vi "RSZVB Get Power Coeficients Default.vi"(8 "error in (no error)":errorcluster {"code" format="%.0x"}, 11 "VISA session":refnum<visa-resource-name>) -> (0 "error out":errorcluster {"code" format="%.0x"}, 1 "Default Coeficients":bool, 3 "dup VISA session":refnum<visa-resource-name>)   [LabVIEW 2011]
doc: "Returns the state of the default power coefficients for frequency converters R&S ZVA-ZxxxE. \n\nNotes:\n\n(1) This command is available for frequency converters with electronic attenuators R&S ZVA-ZxxxE.\n\nRemote-control command(s):\n[SENSe<Ch>:]FREQuency:CONVersion:DEVice:PCOefficient<Port>:DEFault?>"
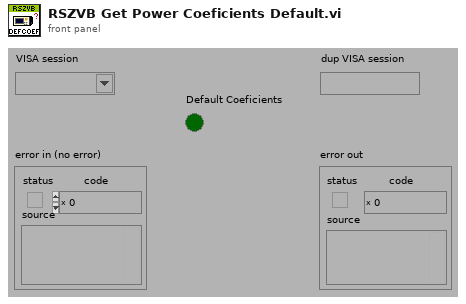
[diagram p1: front panel]
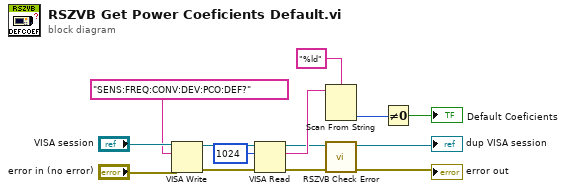
[diagram p0: block diagram]
diagram:
  n1 = VISA Write(VISA resource name="VISA session", write buffer="SENS:FREQ:CONV:DEV:PCO:DEF?", error in (no error)="error in (no error)") -> (VISA resource name out=w10:refnum<visa-resource-name>, error out=w11:errorcluster)  [unwired: 1 out]
  n2 = VISA Read(VISA resource name=w10, byte count=u32 1024, error in (no error)=w11) -> (VISA resource name out=w5:refnum<visa-resource-name>, read buffer=w7:string, error out=w6:errorcluster)  [unwired: 1 out]
  n3 = Scan From String(format string="%ld", input string=w7) -> (output 1=w4:i32)  [unwired: 3 in, 3 out]
  n4 = call "RSZVB Check Error.vi"("error in (no error)"=w6, "VISA session"=w5) -> ("error out"=→"error out":errorcluster, "dup VISA session"=→"dup VISA session":refnum<visa-resource-name>)  [unwired: 8 in]
  n5 = Not Equal To 0?(x=w4) -> (x != 0?=→"Default Coeficients":bool)
